vi "ResultLoadPrompt.vi"(0 "Path":path) -> (1 "selected path":path, 2 "cancel?":bool)   [LabVIEW 2024]
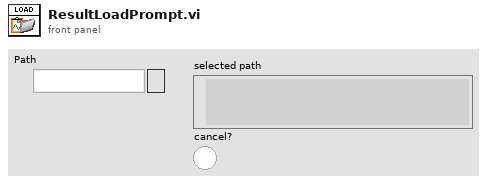
[diagram p1: front panel]
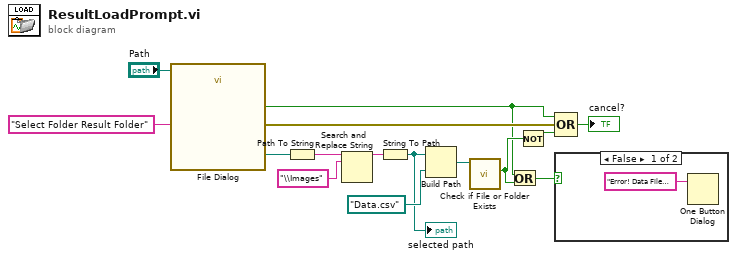
[diagram p0: block diagram]
diagram:
  n1 = call "File Dialog"("start path"="Path", "prompt"="Select Folder Result Folder") -> ("selected path"=w8:path, "cancelled"=w1:bool, "error out"=w15:errorcluster)  [unwired: 10 in, 1 out]
  n2 = Path To String(path=w8) -> (string=w11:string)
  n3 = Search and Replace String(input string=w11, search string="\\Images") -> (result string=w9:string)  [unwired: 6 in, 3 out]
  n4 = String To Path(string=w9) -> (path=w3:path)
  "selected path" <- w3
  n5 = Build Path(base path=w3, name or relative path=path "Data.csv") -> (appended path=w6:path)
  n6 = call <vilib>:"Check if File or Folder Exists.vi"("path"=w6) -> ("file or folder exists?"=w4:bool)  [unwired: 8 in, 2 out]
  n7 = Or(x=w1, y=w4) -> (x .or. y?=w2:bool)
  n8 = Not(x=w4) -> (.not. x?=w5:bool)
  n9 = Compound Arithmetic op=OR(w1, w15, w5) -> (→"cancel?":bool)
  n10 = case shown="False" w2 {
    frame False {
      n11 = One Button Dialog(message="Error! Data File not found in selected folder") -> ()  [unwired: 1 in, 1 out]
    }
    frame True {
    }
  }
